vi "Save File RLT Panel File Name Setup.vi"(0 "File Locations In (Station A)":T4, 1 "Main Washer Control (Station A)":T6={"Appliance Details"={"FileVersionInfo"={"FileVersion"="", "ProductName"="", "InternalName"="", "CompanyName"="", "LegalCopyright"="", "FileDescription"=""}, "Dishwasher Info"={"Open Cup Weight (gm):"=0.0, "Auto Cup Weight (gm):"=0.0, "Detergent-Dish:"="", "Inlet Temperature-Dish:"="", "Cycle Mode-Dish:"="", "Unit Control-Dish:"="", "Manufacturer-Dish:"=""}, "Washer Info"={"Hot Water Temperature (Fahrenheit):"="", "Cold Water Temperature (Fahrenheit):"="", "Capacity (cu.ft):"=0.0, "Initial Cloth Weight:"=0.0, "Cloth Lot:"=0, "Model Family:"="", "Program Name:"="", "Cycle Selection:"="", "Wash Temperature:"="", "Rinse Temperature:"="", "Load Size:"=""}, "File Name Output Array"=[], "Calibration Output Array"=[], "Appliance Common"={"Engineer:"="", "Model Number:"="", "Serial Number:"="", "Comments:"="", "Station ID:"="", "Technician:"="", "TR Number:"="", "Lab ID:"="", "Voltage:"="", "Water Pressure (PSI):"="", "Test Date:"="", "Computer Name:"="", "IP Address:"="", "Ambient RH:"="", "Frequency:"="", "Build:"="", "Filename:"="", "Test Type:"="", "Load Run #:"=0, "Ambient Temperature (F):"="", "File Path:"=path "", "Cycles Per Year"=60}, "Water Heater"={"Heating Mode:"=""}, "Dryer"={"Heat Setting:"="", "Washer Water Temperature (60 ± 5°F):"=60, "Water Hardness (PPM):"=17, "Dryness Setting:"="", "Dryer Type:"="", "Exhaust:"="", "Drying Cycle:"="", "Load Type:"="", "Nominal Load Weight"="", "Dryer Initial IMC Data"={"Measured IMC (lbs)"=7.0, "Actual Initial RMC (%)"=7.0, "RMC (Desired %)"=100.0, "Bone Dry Wt(lbs)"=7.0, "Tolerance(%)"=5.0, "Actual Final RMC (%)"=7.0, "CEF (lbf/kWh)"=0.0, "Minimum Weight (lbf)"=0.0, "Average Weight (lbf)"=0.0, "Maximum Weight (lbf)"=0.0, "Measured IMC In Range?"=FALSE, "Moisture Reduction Factor"=55.5, "Field Use Factor"=1.04, "Empty Dryer Cold Weigth"=0.0, "Energy Standard"=enum."D2-Automatic Dryer", "Weight Cloth (lbs)"=0.0, "Relative Moisture Content (%)"=0.0, "Relative Moisture Content - Avg (%)"=0.0}}}, "Display Data (RLT)"={"Status Color"=0, "Serial Number Display"="", "Cycle Count Display"=0, "Station Label Display"="", "Current Run Start Time Display"=0.0, "Board ID Display"="", "RPM Display"=0, "Current Display"=0.0, "Current Path Display"=path "", "Saving Display"=FALSE, "Unit Type Display"=enum."", "Total Time On Display"=0.0, "UI Button"=FALSE}} {"Display Data (RLT)"."Current Display" format="%.2f"; "Display Data (RLT)"."Cycle Count Display" format="%04d"; "Appliance Details"."Dryer"."Dryer Initial IMC Data"."Maximum Weight (lbf)" format="%03_6g"; "Appliance Details"."Dryer"."Dryer Initial IMC Data"."Average Weight (lbf)" format="%03_6g"; "Appliance Details"."Dryer"."Dryer Initial IMC Data"."Minimum Weight (lbf)" format="%03_6g"; "Appliance Details"."Dryer"."Dryer Initial IMC Data"."CEF (lbf/kWh)" format="%03_6g"; "Appliance Details"."Dryer"."Dryer Initial IMC Data"."Actual Final RMC (%)" format="%03_6g"; "Appliance Details"."Dryer"."Dryer Initial IMC Data"."Tolerance(%)" format="%0#_6g"; "Appliance Details"."Dryer"."Dryer Initial IMC Data"."Bone Dry Wt(lbs)" format="%03_6g"; "Appliance Details"."Dryer"."Dryer Initial IMC Data"."RMC (Desired %)" format="%0#_6g"; "Appliance Details"."Dryer"."Dryer Initial IMC Data"."Actual Initial RMC (%)" format="%03_6g"; "Appliance Details"."Dryer"."Dryer Initial IMC Data"."Measured IMC (lbs)" format="%0#_6g"}, 5 "error in":errorcluster, 6 "RLT Station Type":T13, 11 "Front Panel (Station A)":T2={"Serial Number"="", "Lab ID"="", "TR Number"="", "Unit Type"=enum."", "Source"=228, "Address"=35} {"Address" format="%x"; "Source" format="%x"}) -> (12 "Active Stations":bool[](array[boolean]), 14 "File Locations Out":T4[](array[typedef]), 15 "Main Washer Controls Out":T6[](array[typedef]) {"Display Data (RLT)"."Current Display" format="%.2f"; "Display Data (RLT)"."Cycle Count Display" format="%04d"; "Appliance Details"."Dryer"."Dryer Initial IMC Data"."Maximum Weight (lbf)" format="%03_6g"; "Appliance Details"."Dryer"."Dryer Initial IMC Data"."Average Weight (lbf)" format="%03_6g"; "Appliance Details"."Dryer"."Dryer Initial IMC Data"."Minimum Weight (lbf)" format="%03_6g"; "Appliance Details"."Dryer"."Dryer Initial IMC Data"."CEF (lbf/kWh)" format="%03_6g"; "Appliance Details"."Dryer"."Dryer Initial IMC Data"."Actual Final RMC (%)" format="%03_6g"; "Appliance Details"."Dryer"."Dryer Initial IMC Data"."Tolerance(%)" format="%0#_6g"; "Appliance Details"."Dryer"."Dryer Initial IMC Data"."Bone Dry Wt(lbs)" format="%03_6g"; "Appliance Details"."Dryer"."Dryer Initial IMC Data"."RMC (Desired %)" format="%0#_6g"; "Appliance Details"."Dryer"."Dryer Initial IMC Data"."Actual Initial RMC (%)" format="%03_6g"; "Appliance Details"."Dryer"."Dryer Initial IMC Data"."Measured IMC (lbs)" format="%0#_6g"}, 19 "error out":errorcluster)   [LabVIEW 2016]
uses:
  Public/Type Definitions/Save File Unit Type.ctl
  Save File.lvlib
  Washer HCC/Washer HCC NEWFI/Type Definitions/HCC Filename Setup.ctl
  Type Definition/Save File DOE Data Save Filepaths.ctl
  File Setup.lvlib
  Type Definition/Save File DOE File Path Control.ctl
  <vilib>/Platform/fileVersionInfo.llb/FileVersionInformation.ctl
  Custom Pallet Controls/Custom Pallet String.ctl
  Type Definition/Save File DISH Dishwasher Details.ctl
  Public/Type Definitions/Save File Washer.ctl
  Type Definition/Save File RLT Station Type.ctl
  Public/Type Definitions/Save File Appliance Display.ctl
  Type Definition/DPT IMC Data.ctl
  Washer DOE/Type Definitions/DOE Appliance Common.ctl
  Washer DOE/Type Definitions/DOE Dryer Standard.ctl
panel:
  in  "Station D":T1="StationD"
  in  "Station C":T1="StationC"
  in  "Station B":T1="StationB"
  in  "Station A":T1="StationA"
  in  "Station D Check":bool
  in  "Station C Check":bool
  in  "Station B Check":bool
  in  "Station A Check":bool
  in  "Read Previous (Station D)":bool
  in  "Front Panel (Station D)":T2={"Serial Number"="", "Lab ID"="", "TR Number"="", "Unit Type"=enum."", "Source"=228, "Address"=35} {"Address" format="%x"; "Source" format="%x"}
  in  "Read Previous (Station C)":bool
  in  "Front Panel (Station C)":T2={"Serial Number"="", "Lab ID"="", "TR Number"="", "Unit Type"=enum."", "Source"=228, "Address"=35} {"Address" format="%x"; "Source" format="%x"}
  in  "Read Previous (Station B)":bool
  in  "Front Panel (Station B)":T2={"Serial Number"="", "Lab ID"="", "TR Number"="", "Unit Type"=enum."", "Source"=228, "Address"=35} {"Address" format="%x"; "Source" format="%x"}
  in  "Tab Control":enum32{"Page 1", "Page 2"}(tab)
  in  "File Locations In (Station D)":T4
  in  "File Locations In (Station C)":T4
  in  "File Locations In (Station B)":T4
  in  "Main Washer Control (Station D)":T6={"Appliance Details"={"FileVersionInfo"={"FileVersion"="", "ProductName"="", "InternalName"="", "CompanyName"="", "LegalCopyright"="", "FileDescription"=""}, "Dishwasher Info"={"Open Cup Weight (gm):"=0.0, "Auto Cup Weight (gm):"=0.0, "Detergent-Dish:"="", "Inlet Temperature-Dish:"="", "Cycle Mode-Dish:"="", "Unit Control-Dish:"="", "Manufacturer-Dish:"=""}, "Washer Info"={"Hot Water Temperature (Fahrenheit):"="", "Cold Water Temperature (Fahrenheit):"="", "Capacity (cu.ft):"=0.0, "Initial Cloth Weight:"=0.0, "Cloth Lot:"=0, "Model Family:"="", "Program Name:"="", "Cycle Selection:"="", "Wash Temperature:"="", "Rinse Temperature:"="", "Load Size:"=""}, "File Name Output Array"=[], "Calibration Output Array"=[], "Appliance Common"={"Engineer:"="", "Model Number:"="", "Serial Number:"="", "Comments:"="", "Station ID:"="", "Technician:"="", "TR Number:"="", "Lab ID:"="", "Voltage:"="", "Water Pressure (PSI):"="", "Test Date:"="", "Computer Name:"="", "IP Address:"="", "Ambient RH:"="", "Frequency:"="", "Build:"="", "Filename:"="", "Test Type:"="", "Load Run #:"=0, "Ambient Temperature (F):"="", "File Path:"=path "", "Cycles Per Year"=60}, "Water Heater"={"Heating Mode:"=""}, "Dryer"={"Heat Setting:"="", "Washer Water Temperature (60 ± 5°F):"=60, "Water Hardness (PPM):"=17, "Dryness Setting:"="", "Dryer Type:"="", "Exhaust:"="", "Drying Cycle:"="", "Load Type:"="", "Nominal Load Weight"="", "Dryer Initial IMC Data"={"Measured IMC (lbs)"=7.0, "Actual Initial RMC (%)"=7.0, "RMC (Desired %)"=100.0, "Bone Dry Wt(lbs)"=7.0, "Tolerance(%)"=5.0, "Actual Final RMC (%)"=7.0, "CEF (lbf/kWh)"=0.0, "Minimum Weight (lbf)"=0.0, "Average Weight (lbf)"=0.0, "Maximum Weight (lbf)"=0.0, "Measured IMC In Range?"=FALSE, "Moisture Reduction Factor"=55.5, "Field Use Factor"=1.04, "Empty Dryer Cold Weigth"=0.0, "Energy Standard"=enum."D2-Automatic Dryer", "Weight Cloth (lbs)"=0.0, "Relative Moisture Content (%)"=0.0, "Relative Moisture Content - Avg (%)"=0.0}}}, "Display Data (RLT)"={"Status Color"=0, "Serial Number Display"="", "Cycle Count Display"=0, "Station Label Display"="", "Current Run Start Time Display"=0.0, "Board ID Display"="", "RPM Display"=0, "Current Display"=0.0, "Current Path Display"=path "", "Saving Display"=FALSE, "Unit Type Display"=enum."", "Total Time On Display"=0.0, "UI Button"=FALSE}} {"Display Data (RLT)"."Current Display" format="%.2f"; "Display Data (RLT)"."Cycle Count Display" format="%04d"; "Appliance Details"."Dryer"."Dryer Initial IMC Data"."Maximum Weight (lbf)" format="%03_6g"; "Appliance Details"."Dryer"."Dryer Initial IMC Data"."Average Weight (lbf)" format="%03_6g"; "Appliance Details"."Dryer"."Dryer Initial IMC Data"."Minimum Weight (lbf)" format="%03_6g"; "Appliance Details"."Dryer"."Dryer Initial IMC Data"."CEF (lbf/kWh)" format="%03_6g"; "Appliance Details"."Dryer"."Dryer Initial IMC Data"."Actual Final RMC (%)" format="%03_6g"; "Appliance Details"."Dryer"."Dryer Initial IMC Data"."Tolerance(%)" format="%0#_6g"; "Appliance Details"."Dryer"."Dryer Initial IMC Data"."Bone Dry Wt(lbs)" format="%03_6g"; "Appliance Details"."Dryer"."Dryer Initial IMC Data"."RMC (Desired %)" format="%0#_6g"; "Appliance Details"."Dryer"."Dryer Initial IMC Data"."Actual Initial RMC (%)" format="%03_6g"; "Appliance Details"."Dryer"."Dryer Initial IMC Data"."Measured IMC (lbs)" format="%0#_6g"}
  in  "Main Washer Control (Station C)":T6={"Appliance Details"={"FileVersionInfo"={"FileVersion"="", "ProductName"="", "InternalName"="", "CompanyName"="", "LegalCopyright"="", "FileDescription"=""}, "Dishwasher Info"={"Open Cup Weight (gm):"=0.0, "Auto Cup Weight (gm):"=0.0, "Detergent-Dish:"="", "Inlet Temperature-Dish:"="", "Cycle Mode-Dish:"="", "Unit Control-Dish:"="", "Manufacturer-Dish:"=""}, "Washer Info"={"Hot Water Temperature (Fahrenheit):"="", "Cold Water Temperature (Fahrenheit):"="", "Capacity (cu.ft):"=0.0, "Initial Cloth Weight:"=0.0, "Cloth Lot:"=0, "Model Family:"="", "Program Name:"="", "Cycle Selection:"="", "Wash Temperature:"="", "Rinse Temperature:"="", "Load Size:"=""}, "File Name Output Array"=[], "Calibration Output Array"=[], "Appliance Common"={"Engineer:"="", "Model Number:"="", "Serial Number:"="", "Comments:"="", "Station ID:"="", "Technician:"="", "TR Number:"="", "Lab ID:"="", "Voltage:"="", "Water Pressure (PSI):"="", "Test Date:"="", "Computer Name:"="", "IP Address:"="", "Ambient RH:"="", "Frequency:"="", "Build:"="", "Filename:"="", "Test Type:"="", "Load Run #:"=0, "Ambient Temperature (F):"="", "File Path:"=path "", "Cycles Per Year"=60}, "Water Heater"={"Heating Mode:"=""}, "Dryer"={"Heat Setting:"="", "Washer Water Temperature (60 ± 5°F):"=60, "Water Hardness (PPM):"=17, "Dryness Setting:"="", "Dryer Type:"="", "Exhaust:"="", "Drying Cycle:"="", "Load Type:"="", "Nominal Load Weight"="", "Dryer Initial IMC Data"={"Measured IMC (lbs)"=7.0, "Actual Initial RMC (%)"=7.0, "RMC (Desired %)"=100.0, "Bone Dry Wt(lbs)"=7.0, "Tolerance(%)"=5.0, "Actual Final RMC (%)"=7.0, "CEF (lbf/kWh)"=0.0, "Minimum Weight (lbf)"=0.0, "Average Weight (lbf)"=0.0, "Maximum Weight (lbf)"=0.0, "Measured IMC In Range?"=FALSE, "Moisture Reduction Factor"=55.5, "Field Use Factor"=1.04, "Empty Dryer Cold Weigth"=0.0, "Energy Standard"=enum."D2-Automatic Dryer", "Weight Cloth (lbs)"=0.0, "Relative Moisture Content (%)"=0.0, "Relative Moisture Content - Avg (%)"=0.0}}}, "Display Data (RLT)"={"Status Color"=0, "Serial Number Display"="", "Cycle Count Display"=0, "Station Label Display"="", "Current Run Start Time Display"=0.0, "Board ID Display"="", "RPM Display"=0, "Current Display"=0.0, "Current Path Display"=path "", "Saving Display"=FALSE, "Unit Type Display"=enum."", "Total Time On Display"=0.0, "UI Button"=FALSE}} {"Display Data (RLT)"."Current Display" format="%.2f"; "Display Data (RLT)"."Cycle Count Display" format="%04d"; "Appliance Details"."Dryer"."Dryer Initial IMC Data"."Maximum Weight (lbf)" format="%03_6g"; "Appliance Details"."Dryer"."Dryer Initial IMC Data"."Average Weight (lbf)" format="%03_6g"; "Appliance Details"."Dryer"."Dryer Initial IMC Data"."Minimum Weight (lbf)" format="%03_6g"; "Appliance Details"."Dryer"."Dryer Initial IMC Data"."CEF (lbf/kWh)" format="%03_6g"; "Appliance Details"."Dryer"."Dryer Initial IMC Data"."Actual Final RMC (%)" format="%03_6g"; "Appliance Details"."Dryer"."Dryer Initial IMC Data"."Tolerance(%)" format="%0#_6g"; "Appliance Details"."Dryer"."Dryer Initial IMC Data"."Bone Dry Wt(lbs)" format="%03_6g"; "Appliance Details"."Dryer"."Dryer Initial IMC Data"."RMC (Desired %)" format="%0#_6g"; "Appliance Details"."Dryer"."Dryer Initial IMC Data"."Actual Initial RMC (%)" format="%03_6g"; "Appliance Details"."Dryer"."Dryer Initial IMC Data"."Measured IMC (lbs)" format="%0#_6g"}
  in  "Main Washer Control (Station B)":T6={"Appliance Details"={"FileVersionInfo"={"FileVersion"="", "ProductName"="", "InternalName"="", "CompanyName"="", "LegalCopyright"="", "FileDescription"=""}, "Dishwasher Info"={"Open Cup Weight (gm):"=0.0, "Auto Cup Weight (gm):"=0.0, "Detergent-Dish:"="", "Inlet Temperature-Dish:"="", "Cycle Mode-Dish:"="", "Unit Control-Dish:"="", "Manufacturer-Dish:"=""}, "Washer Info"={"Hot Water Temperature (Fahrenheit):"="", "Cold Water Temperature (Fahrenheit):"="", "Capacity (cu.ft):"=0.0, "Initial Cloth Weight:"=0.0, "Cloth Lot:"=0, "Model Family:"="", "Program Name:"="", "Cycle Selection:"="", "Wash Temperature:"="", "Rinse Temperature:"="", "Load Size:"=""}, "File Name Output Array"=[], "Calibration Output Array"=[], "Appliance Common"={"Engineer:"="", "Model Number:"="", "Serial Number:"="", "Comments:"="", "Station ID:"="", "Technician:"="", "TR Number:"="", "Lab ID:"="", "Voltage:"="", "Water Pressure (PSI):"="", "Test Date:"="", "Computer Name:"="", "IP Address:"="", "Ambient RH:"="", "Frequency:"="", "Build:"="", "Filename:"="", "Test Type:"="", "Load Run #:"=0, "Ambient Temperature (F):"="", "File Path:"=path "", "Cycles Per Year"=60}, "Water Heater"={"Heating Mode:"=""}, "Dryer"={"Heat Setting:"="", "Washer Water Temperature (60 ± 5°F):"=60, "Water Hardness (PPM):"=17, "Dryness Setting:"="", "Dryer Type:"="", "Exhaust:"="", "Drying Cycle:"="", "Load Type:"="", "Nominal Load Weight"="", "Dryer Initial IMC Data"={"Measured IMC (lbs)"=7.0, "Actual Initial RMC (%)"=7.0, "RMC (Desired %)"=100.0, "Bone Dry Wt(lbs)"=7.0, "Tolerance(%)"=5.0, "Actual Final RMC (%)"=7.0, "CEF (lbf/kWh)"=0.0, "Minimum Weight (lbf)"=0.0, "Average Weight (lbf)"=0.0, "Maximum Weight (lbf)"=0.0, "Measured IMC In Range?"=FALSE, "Moisture Reduction Factor"=55.5, "Field Use Factor"=1.04, "Empty Dryer Cold Weigth"=0.0, "Energy Standard"=enum."D2-Automatic Dryer", "Weight Cloth (lbs)"=0.0, "Relative Moisture Content (%)"=0.0, "Relative Moisture Content - Avg (%)"=0.0}}}, "Display Data (RLT)"={"Status Color"=0, "Serial Number Display"="", "Cycle Count Display"=0, "Station Label Display"="", "Current Run Start Time Display"=0.0, "Board ID Display"="", "RPM Display"=0, "Current Display"=0.0, "Current Path Display"=path "", "Saving Display"=FALSE, "Unit Type Display"=enum."", "Total Time On Display"=0.0, "UI Button"=FALSE}} {"Display Data (RLT)"."Current Display" format="%.2f"; "Display Data (RLT)"."Cycle Count Display" format="%04d"; "Appliance Details"."Dryer"."Dryer Initial IMC Data"."Maximum Weight (lbf)" format="%03_6g"; "Appliance Details"."Dryer"."Dryer Initial IMC Data"."Average Weight (lbf)" format="%03_6g"; "Appliance Details"."Dryer"."Dryer Initial IMC Data"."Minimum Weight (lbf)" format="%03_6g"; "Appliance Details"."Dryer"."Dryer Initial IMC Data"."CEF (lbf/kWh)" format="%03_6g"; "Appliance Details"."Dryer"."Dryer Initial IMC Data"."Actual Final RMC (%)" format="%03_6g"; "Appliance Details"."Dryer"."Dryer Initial IMC Data"."Tolerance(%)" format="%0#_6g"; "Appliance Details"."Dryer"."Dryer Initial IMC Data"."Bone Dry Wt(lbs)" format="%03_6g"; "Appliance Details"."Dryer"."Dryer Initial IMC Data"."RMC (Desired %)" format="%0#_6g"; "Appliance Details"."Dryer"."Dryer Initial IMC Data"."Actual Initial RMC (%)" format="%03_6g"; "Appliance Details"."Dryer"."Dryer Initial IMC Data"."Measured IMC (lbs)" format="%0#_6g"}
  in  "Read Previous (Station A)":bool
  in  "Tab Control 2":enum32{"Input Data", "Error Data"}(tab)
  in  "Complete":bool
  # "OR"
  # "OR"
  # "OR"
  # "OR"
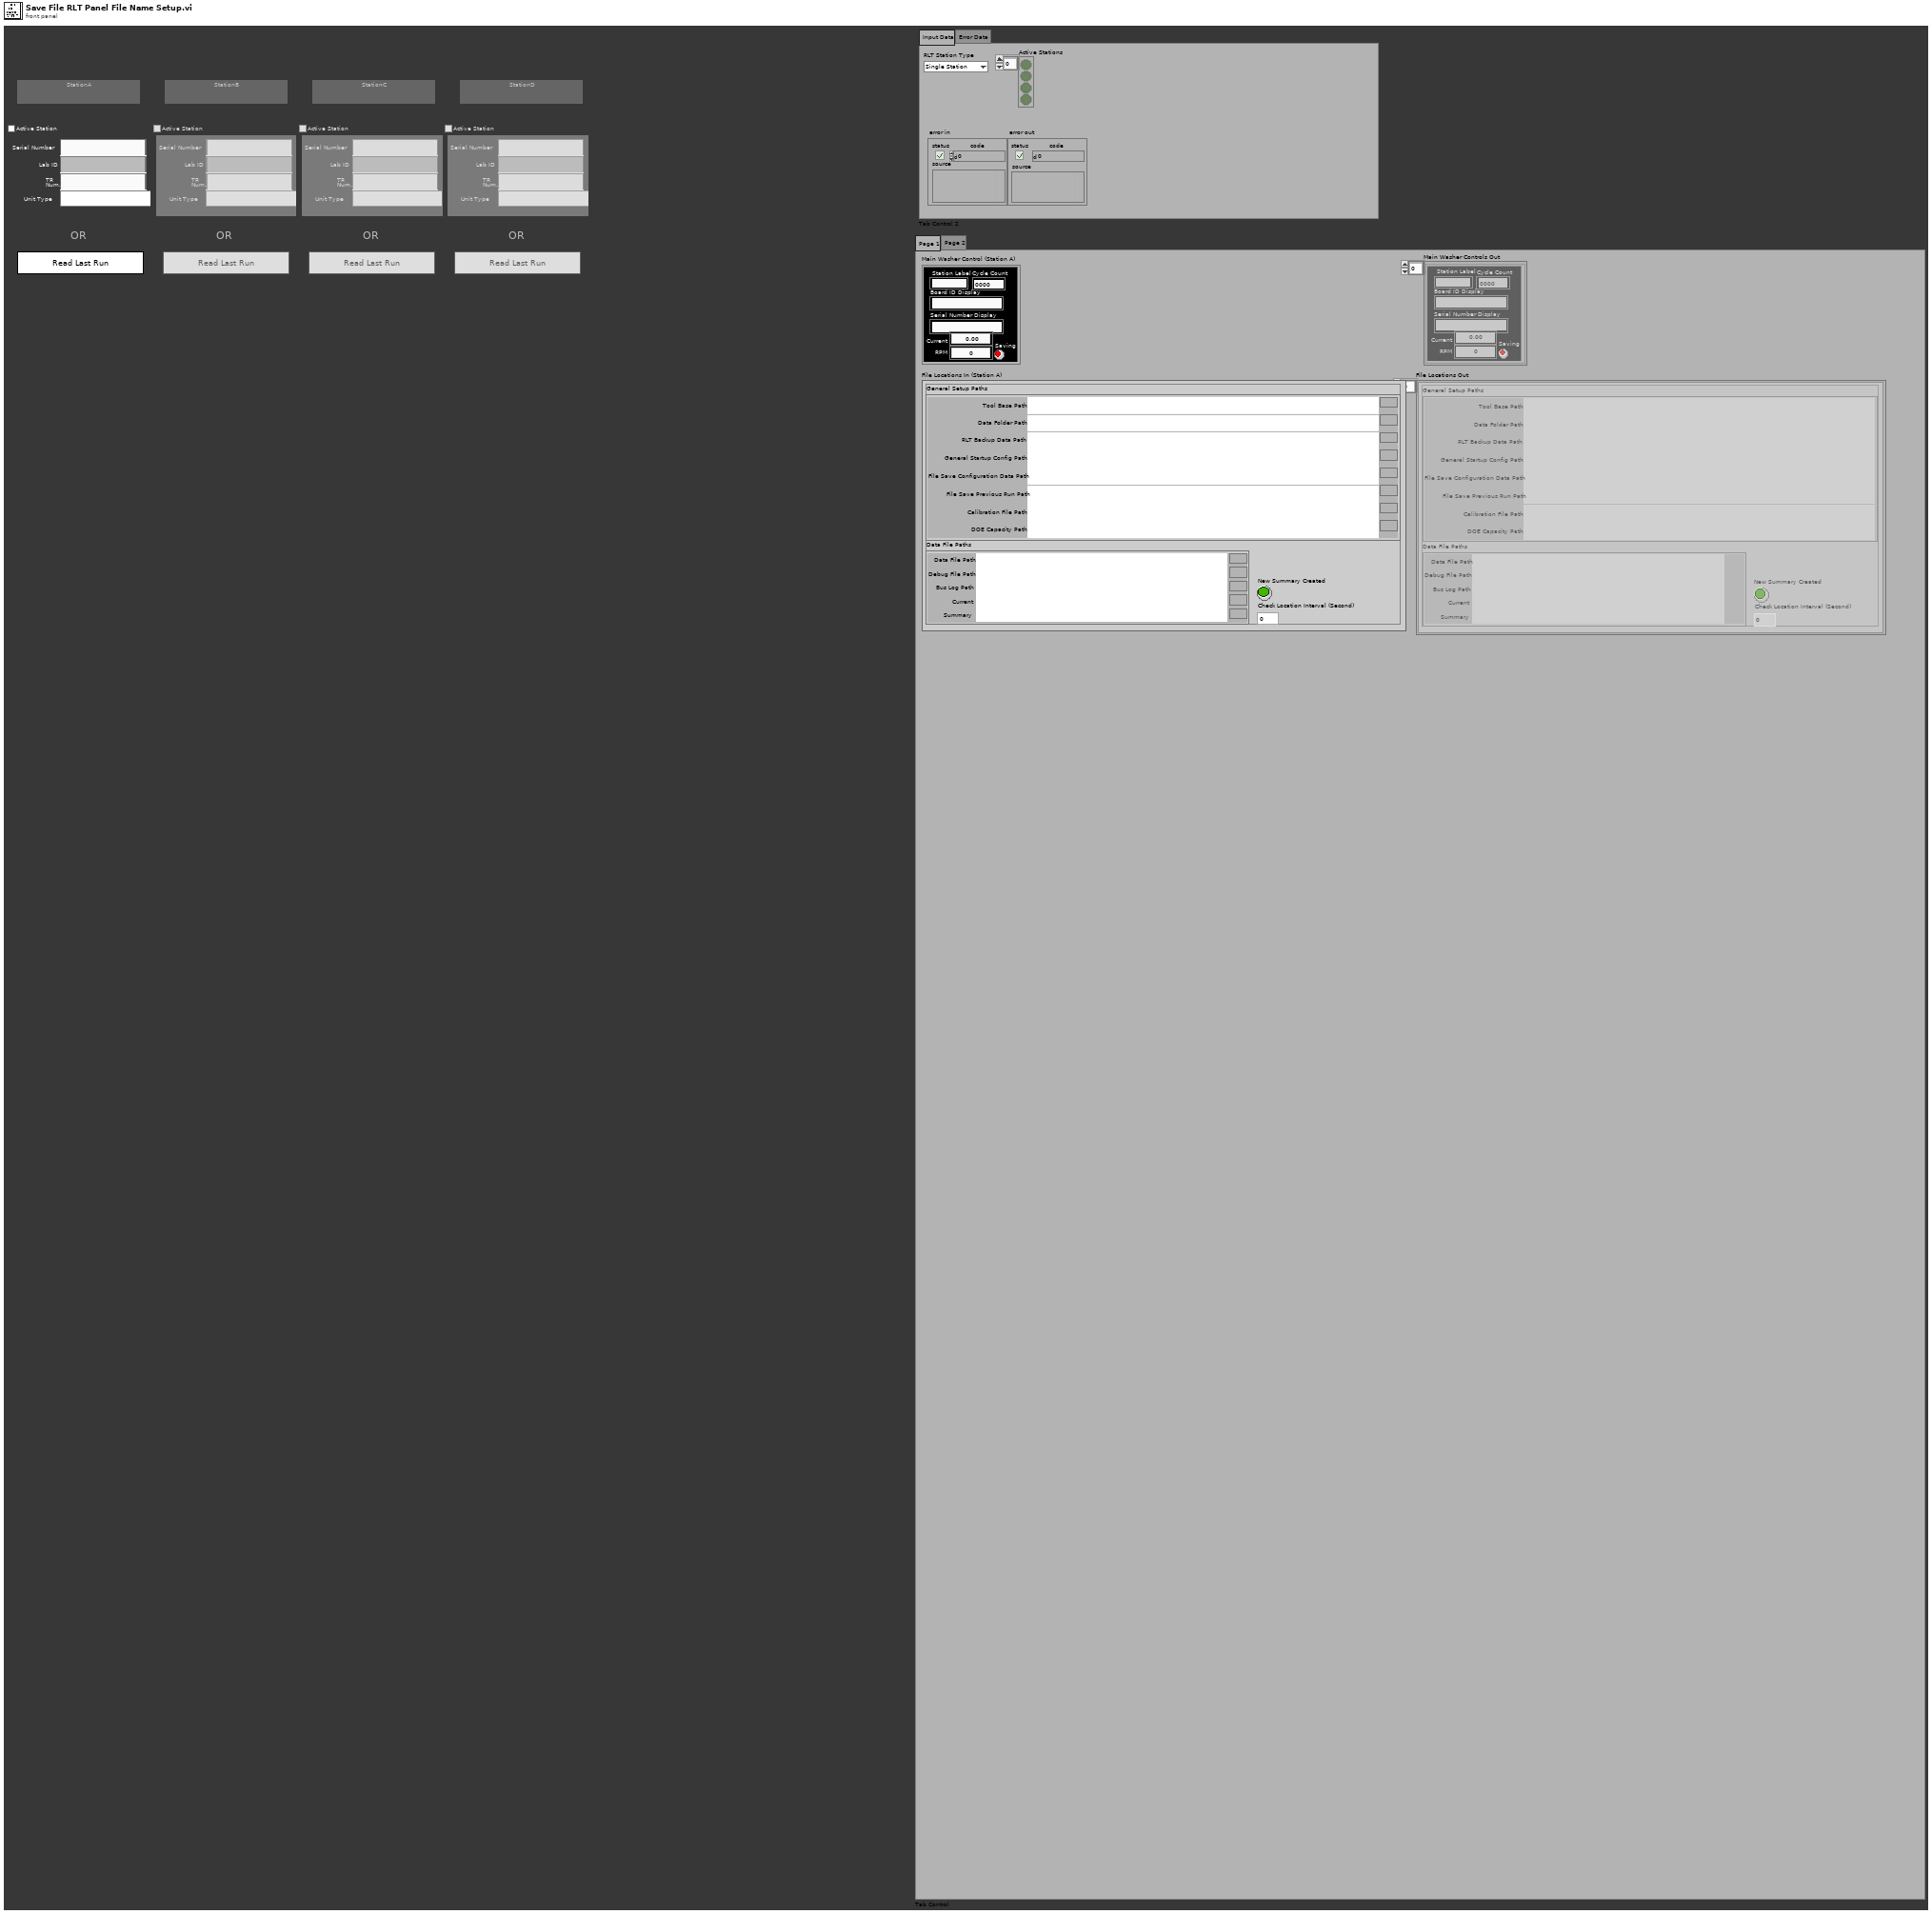
[diagram p1: front panel]
types:
  T1 = typedef "Custom Pallet String.ctl" = string
  T2 = typedef "HCC Filename Setup.ctl" = cluster{"Serial Number":string, "Lab ID":string, "TR Number":string, "Unit Type":T3, "Source":u8, "Address":u8}
  T3 = typedef "Save File.lvlib/Save File Unit Type.ctl" = enum32{"", "Viper", "Hawk", "2015"}
  T4 = typedef "File Setup.lvlib/Save File DOE File Path Control.ctl" = cluster{"General Setup Paths":cluster{"Calibration File Path":path, "DOE Capacity Path":path, "Data Folder Path":path, "RLT Backup Data Path":path, "Tool Base Path":path, "General Startup Config Path":path, "File Save Previous Run Path":path, "File Save Configuration Data Path":path}, "Data File Paths":T5, "New Summary Created":bool, "Check Location Interval (Second)":i32}
  T5 = typedef "File Setup.lvlib/Save File DOE Data Save Filepaths.ctl" = cluster{"Data File Path":path, "Debug File Path":path, "Bus Log Path":path, "Current":path, "Summary":path}
  T6 = typedef "Save File.lvlib/Save File Washer.ctl" = cluster{"Appliance Details":T7, "Display Data (RLT)":T12}
  T7 = typedef "File Setup.lvlib/Save File DISH Dishwasher Details.ctl" = cluster{"FileVersionInfo":T8, "Dishwasher Info":cluster{"Open Cup Weight (gm):":dbl, "Auto Cup Weight (gm):":dbl, "Detergent-Dish:":string, "Inlet Temperature-Dish:":string, "Cycle Mode-Dish:":string, "Unit Control-Dish:":string, "Manufacturer-Dish:":string}, "Washer Info":cluster{"Hot Water Temperature (Fahrenheit):":string, "Cold Water Temperature (Fahrenheit):":string, "Capacity (cu.ft):":dbl, "Initial Cloth Weight:":dbl, "Cloth Lot:":i32, "Model Family:":string, "Program Name:":string, "Cycle Selection:":string, "Wash Temperature:":string, "Rinse Temperature:":string, "Load Size:":string}, "File Name Output Array":string[][], "Calibration Output Array":string[][], "Appliance Common":T9, "Water Heater":cluster{"Heating Mode:":string}, "Dryer":cluster{"Heat Setting:":T1, "Washer Water Temperature (60 ± 5°F):":u16, "Water Hardness (PPM):":u16, "Dryness Setting:":T1, "Dryer Type:":string, "Exhaust:":string, "Drying Cycle:":string, "Load Type:":string, "Nominal Load Weight":string, "Dryer Initial IMC Data":T10}}
  T8 = typedef "FileVersionInformation.ctl" = cluster{"FileVersion":string, "ProductName":string, "InternalName":string, "CompanyName":string, "LegalCopyright":string, "FileDescription":string}
  T9 = typedef "DOE Appliance Common.ctl" = cluster{"Engineer:":string, "Model Number:":string, "Serial Number:":string, "Comments:":string, "Station ID:":string, "Technician:":string, "TR Number:":string, "Lab ID:":string, "Voltage:":string, "Water Pressure (PSI):":string, "Test Date:":string, "Computer Name:":string, "IP Address:":string, "Ambient RH:":string, "Frequency:":string, "Build:":string, "Filename:":string, "Test Type:":string, "Load Run #:":i32, "Ambient Temperature (F):":string, "File Path:":path, "Cycles Per Year":u32}
  T10 = typedef "DPT IMC Data.ctl" = cluster{"Measured IMC (lbs)":dbl, "Actual Initial RMC (%)":dbl, "RMC (Desired %)":dbl, "Bone Dry Wt(lbs)":dbl, "Tolerance(%)":dbl, "Actual Final RMC (%)":dbl, "CEF (lbf/kWh)":dbl, "Minimum Weight (lbf)":dbl, "Average Weight (lbf)":dbl, "Maximum Weight (lbf)":dbl, "Measured IMC In Range?":bool, "Moisture Reduction Factor":dbl, "Field Use Factor":dbl, "Empty Dryer Cold Weigth":dbl, "Energy Standard":T11, "Weight Cloth (lbs)":dbl, "Relative Moisture Content (%)":dbl, "Relative Moisture Content - Avg (%)":dbl}
  T11 = typedef "DOE Dryer Standard.ctl" = enum16{"D2-Automatic Dryer", "D2-Timer Dryer", "D1-Automatic Dryer", "D1-Timer Dryer", "Other"}
  T12 = typedef "Save File Appliance Display.ctl" = cluster{"Status Color":u32, "Serial Number Display":string, "Cycle Count Display":i32, "Station Label Display":string, "Current Run Start Time Display":dbl, "Board ID Display":string, "RPM Display":u32, "Current Display":dbl, "Current Path Display":path, "Saving Display":bool, "Unit Type Display":T3, "Total Time On Display":dbl, "UI Button":bool}
  T13 = typedef "Save File RLT Station Type.ctl" = enum16{"Single Station", "Four Stations"}
  T14 = enum8{"Enabled", "Disabled", "Disabled and Grayed Out"}
  T15 = enum32{"invalid app kind", "Development System", "Run Time System", "Student Edition", "Embedded LabVIEW", "Evaluation", "Custom"}
  T16 = enum32{"Invalid", "Standard", "Closed", "Hidden", "Minimized", "Maximized"}
  T17 = cluster{"Core":cluster{"Current VI Reference":refnum<vi>, "Close Panel on Exit?":bool}, "Main Washer Control (Station A)":T6, "Main Washer Control (Station B)":T6, "Main Washer Control (Station C)":T6, "Main Washer Control (Station D)":T6, "Front Panel (Station A)":T2, "Front Panel (Station B)":T2, "Front Panel (Station C)":T2, "Front Panel (Station D)":T2, "File Locations In (Station A)":T4, "File Locations In (Station B)":T4, "File Locations In (Station C)":T4, "File Locations In (Station D)":T4, "Active Stations":bool[], "RLT Station Type":T13}
  T18 = cluster{"Current VI Reference":refnum<vi>, "Close Panel on Exit?":bool}
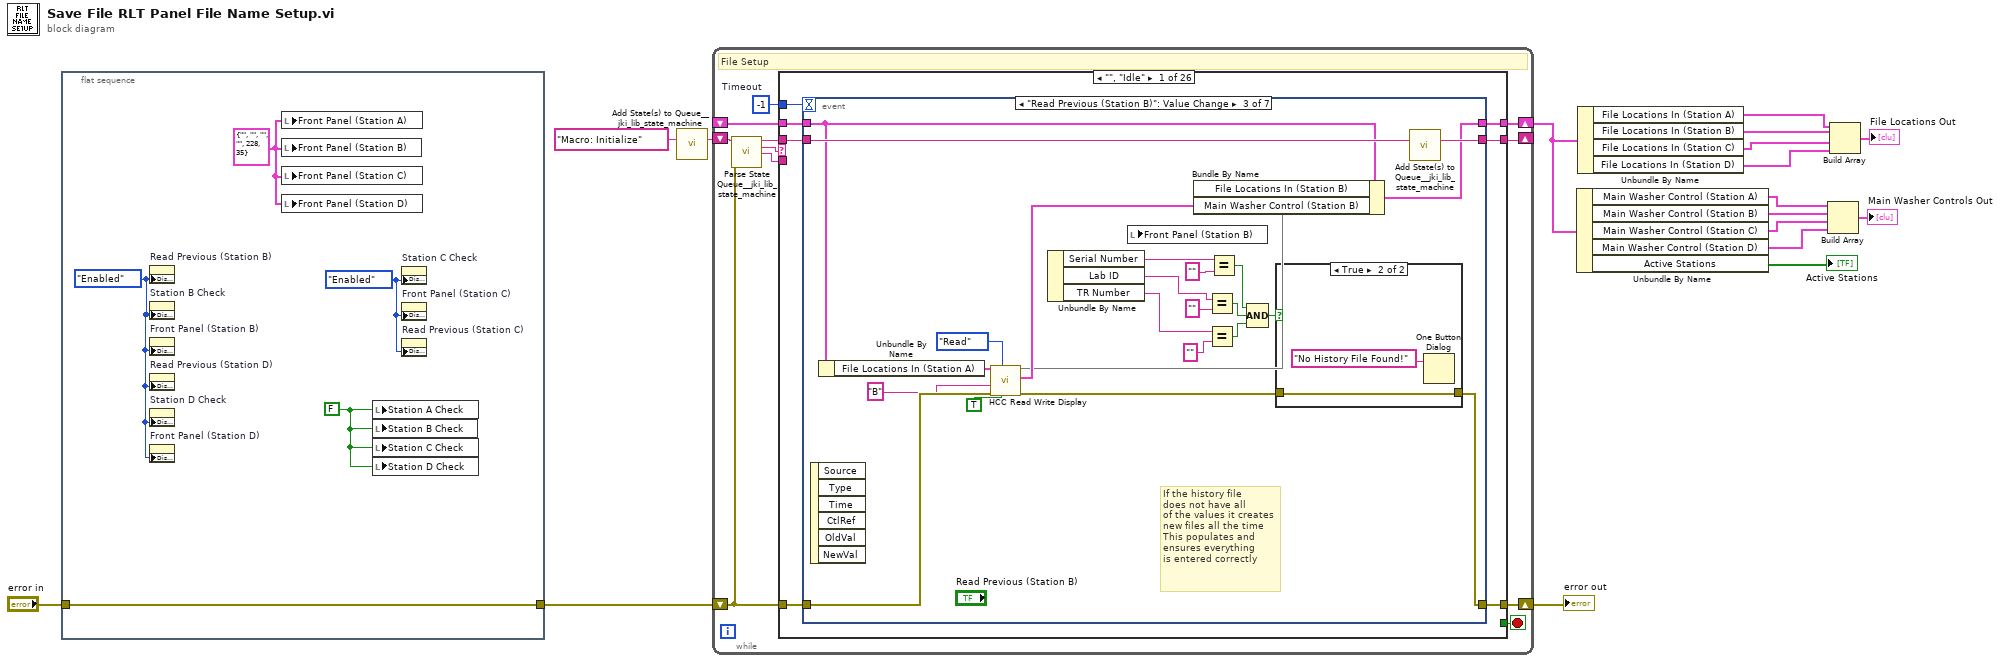
[diagram p0: block diagram]
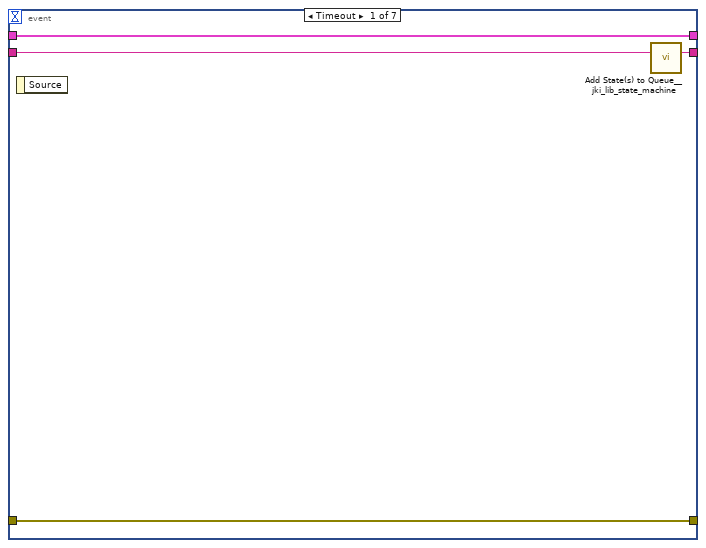
[diagram p2: hidden frame]
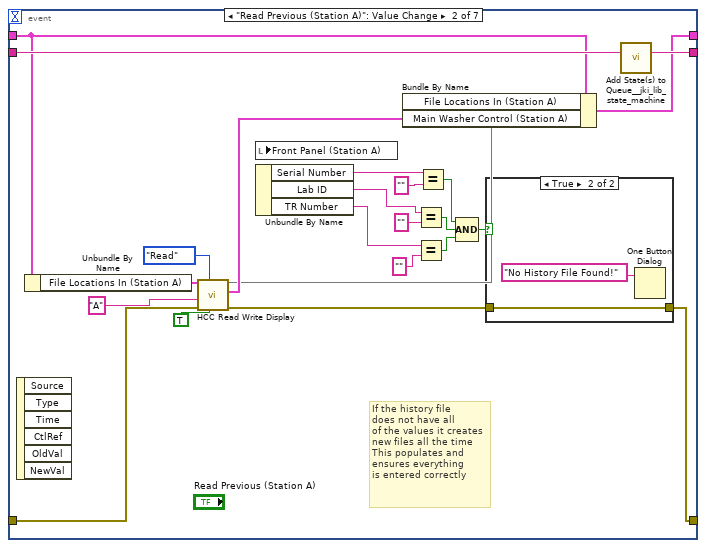
[diagram p3: hidden frame]
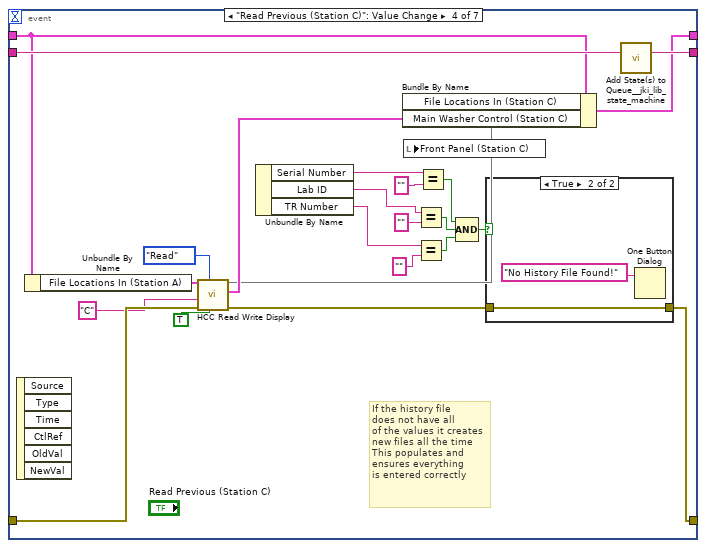
[diagram p6: hidden frame]
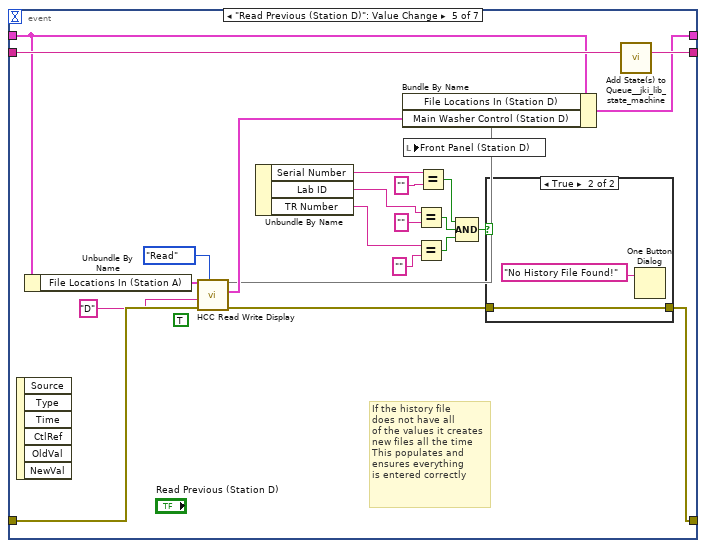
[diagram p8: hidden frame]
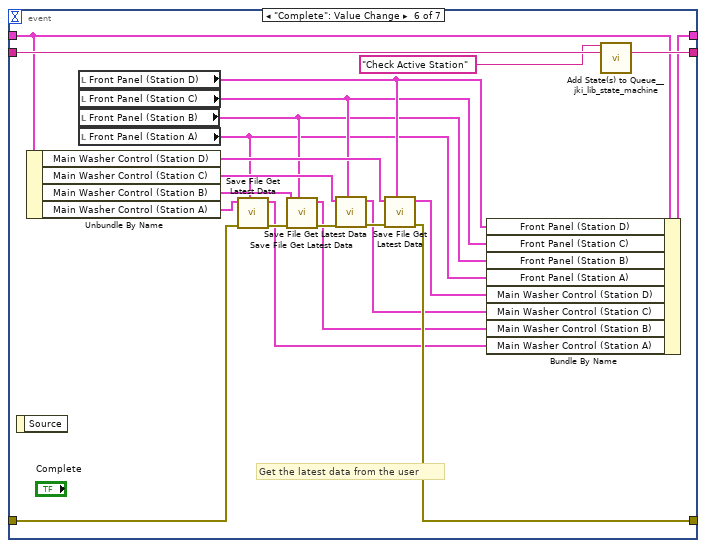
[diagram p10: hidden frame]
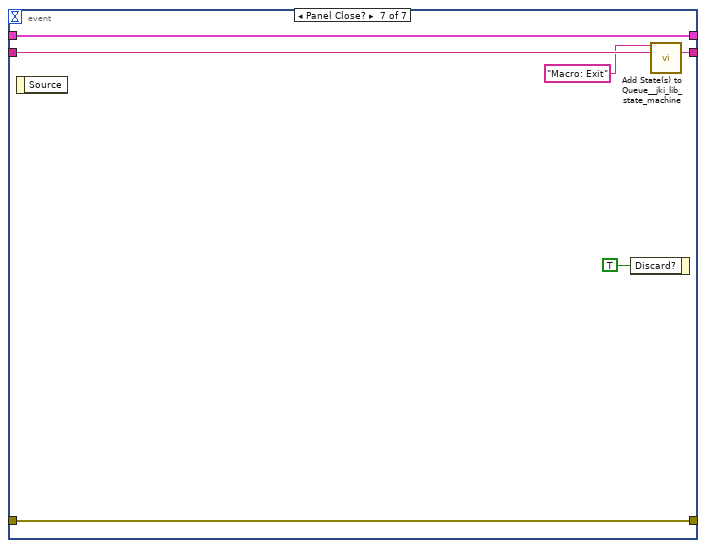
[diagram p11: hidden frame]
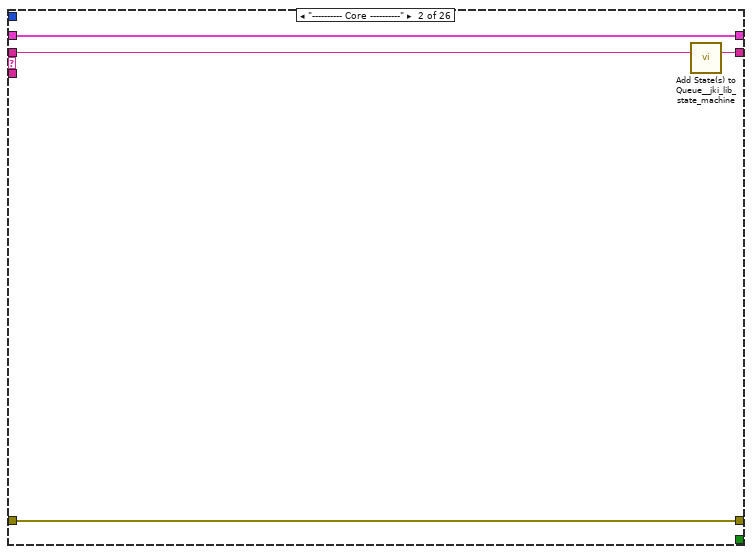
[diagram p12: hidden frame]
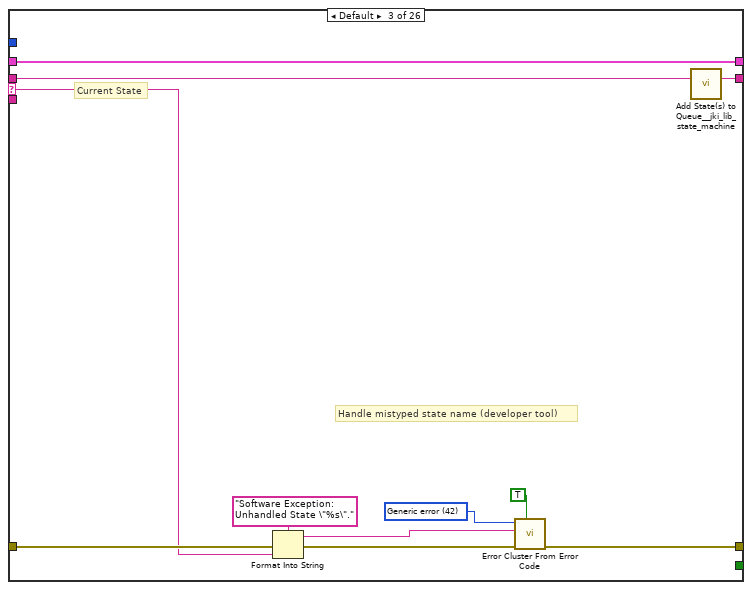
[diagram p13: hidden frame]
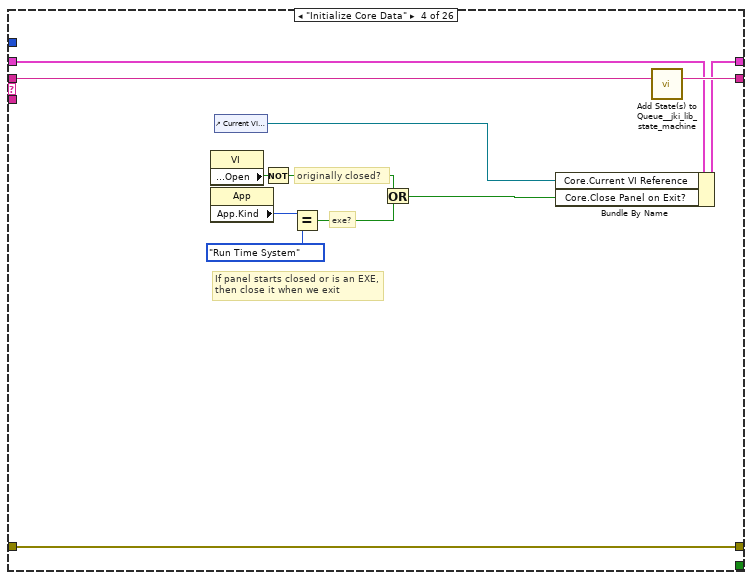
[diagram p14: hidden frame]
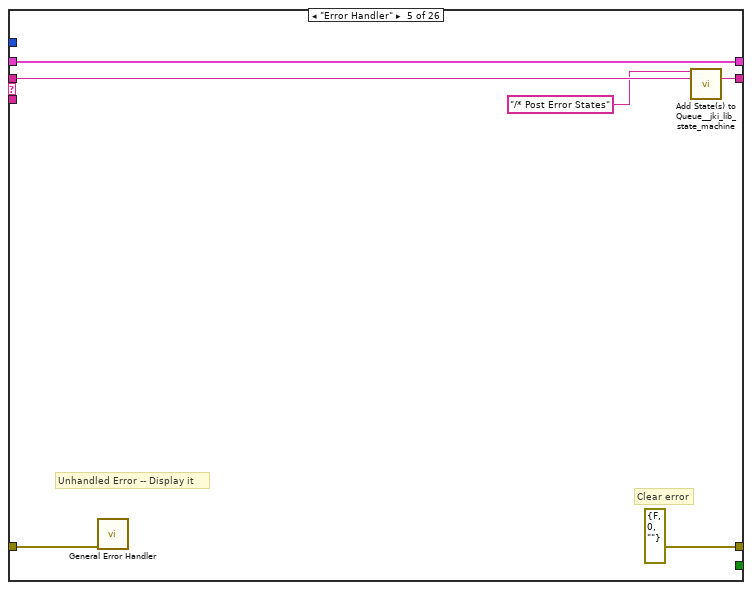
[diagram p15: hidden frame]
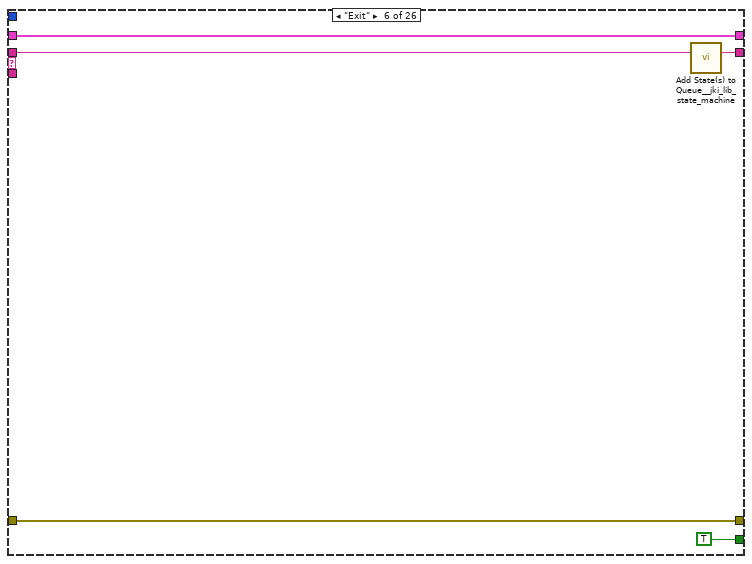
[diagram p16: hidden frame]
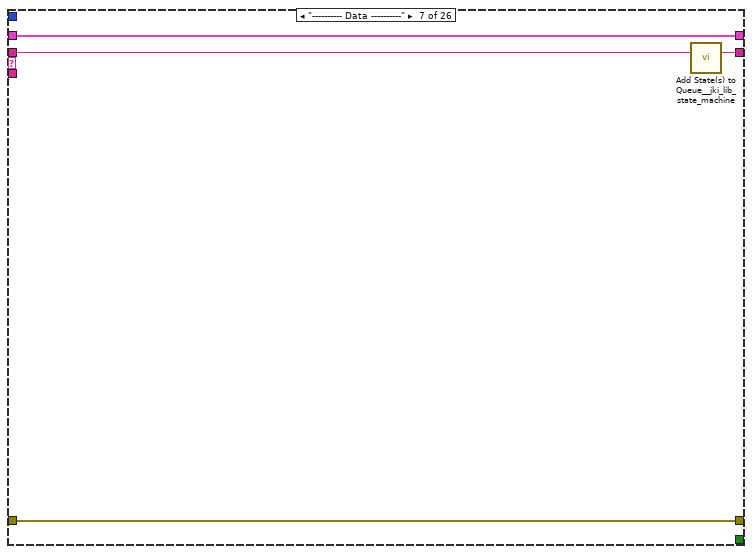
[diagram p17: hidden frame]
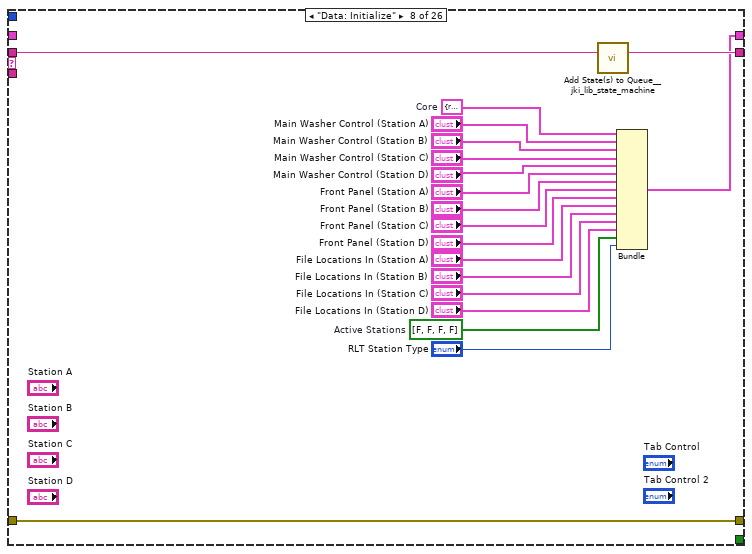
[diagram p18: hidden frame]
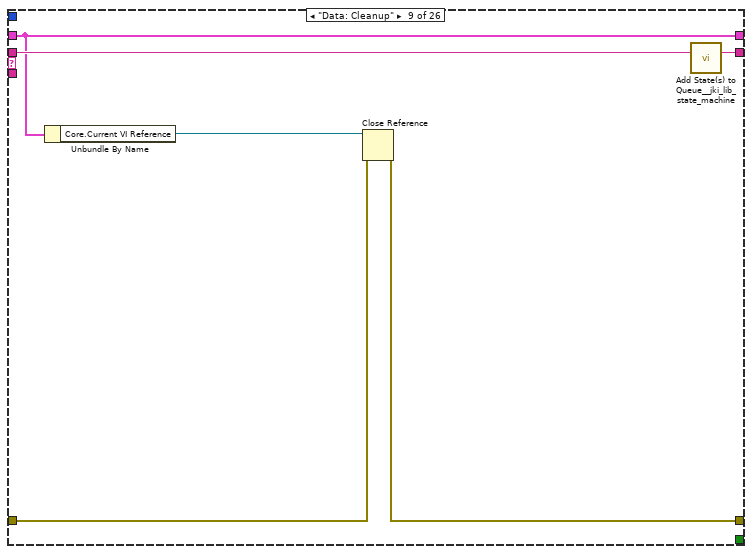
[diagram p19: hidden frame]
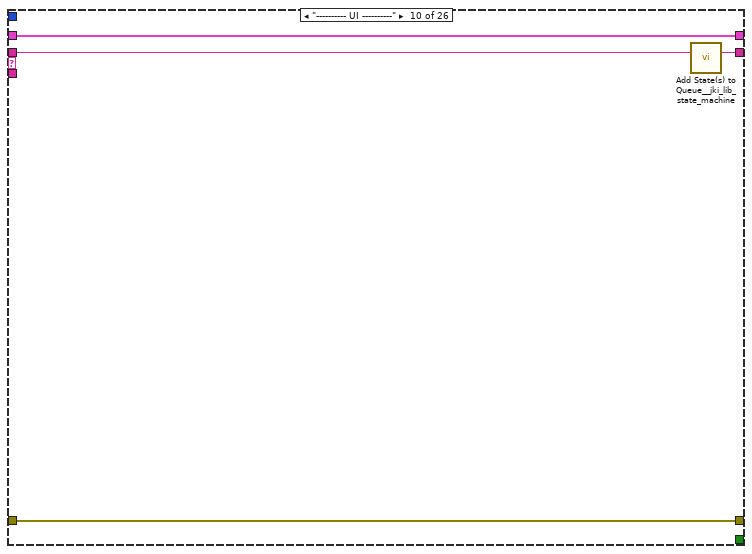
[diagram p20: hidden frame]
diagram:
  n1 = flat-sequence {
    tunnel: "error in" -> [w20]
    tunnel: [w20] -> w2
    frame #0 {
      w18 = T2 {"Serial Number"="", "Lab ID"="", "TR Number"="", "Unit Type"=enum."", "Source"=228, "Address"=35} ("Front Panel (Station A)")
      w19 = FALSE ("Station A Check")
      w22 = T14."Enabled" ("Disabled")
      w21 = T14."Enabled" ("Disabled")
      n2 = property on="Read Previous (Station B)" class="Bool"("DisabledEnum"=w21) -> ()  [unwired: 2 in, 2 out]
      n3 = property on="Station B Check" class="Bool (strict)"("DisabledEnum"=w21) -> ()  [unwired: 2 in, 2 out]
      n4 = property on="Front Panel (Station B)" class="Clust (strict)"("DisabledEnum"=w21) -> ()  [unwired: 2 in, 2 out]
      n5 = property on="Read Previous (Station D)" class="Bool"("DisabledEnum"=w21) -> ()  [unwired: 2 in, 2 out]
      n6 = property on="Station D Check" class="Bool (strict)"("DisabledEnum"=w21) -> ()  [unwired: 2 in, 2 out]
      n7 = property on="Front Panel (Station D)" class="Clust (strict)"("DisabledEnum"=w21) -> ()  [unwired: 2 in, 2 out]
      n8 = local write "Front Panel (Station A)"(w18) -> ()
      n9 = local write "Front Panel (Station B)"(w18) -> ()
      n10 = local write "Front Panel (Station C)"(w18) -> ()
      n11 = local write "Front Panel (Station D)"(w18) -> ()
      n12 = local write "Station A Check"(w19) -> ()
      n13 = local write "Station B Check"(w19) -> ()
      n14 = local write "Station C Check"(w19) -> ()
      n15 = local write "Station D Check"(w19) -> ()
      n16 = property on="Station C Check" class="Bool (strict)"("DisabledEnum"=w22) -> ()  [unwired: 2 in, 2 out]
      n17 = property on="Front Panel (Station C)" class="Clust (strict)"("DisabledEnum"=w22) -> ()  [unwired: 2 in, 2 out]
      n18 = property on="Read Previous (Station C)" class="Bool"("DisabledEnum"=w22) -> ()  [unwired: 2 in, 2 out]
    }
  }
  n19 = call <vilib>:"Add State(s) to Queue__jki_lib_state_machine.vi"("State(s) in (\"\")"="Macro: Initialize") -> ("States Out"=w17:string)  [unwired: 14 in]
  n20 = while "File Setup" {
    shift-right: [w26] -> w14
    shift-left: _ -> [w25]
    shift-right: [w29] -> w16
    shift-left: w2 -> [w23]
    shift-right: [w28] -> _
    shift-left: w17 -> [w30]
    stop <- w27 stop-if-true
    w24 = -1  # Timeout
    # "File Setup"
    n21 = call <vilib>:"Parse State Queue__jki_lib_state_machine.vi"("State Queue"=w30, "Error In (no error)"=w23) -> ("Remaining States"=w32:string, "Current State"=w33:string, "Arguments"=w31:string)  [unwired: 11 in]
    n22 = case shown="\"\", \"Idle\"" w33 {
      selector: w33 -> [_ _ w180 _ _ _ _ _ _ _ _ _ _ _ _ _ _ _ _ _ _ _ _ _ _ _]
      tunnel: w32 -> [w40 w179 w184 w202 w208 w213 w217 w236 w242 w246 w252 w262 w273 w299 w304 w314 w318 w330 w343 w356 w369 w382 w400 w415 w430 w445]
      tunnel: w31 -> [_ _ _ _ _ _ _ _ _ _ _ w257 w267 _ _ _ _ _ _ _ _ _ _ _ _ _]
      tunnel: w25 -> [w38 w176 w182 w193 w205 w211 w214 _ w237 w243 w250 w260 w269 w296 w301 w311 w315 w322 w337 w351 w364 w379 w394 w409 w424 w439]
      tunnel: [w37 w177 w186 w199 errorcluster {"status"=FALSE, "code"=0, "source"=""} ("error out") w210 w215 w233 w238 w244 w248 w258 w270 w297 w302 w312 w316 w328 w338 w347 w365 w376 w395 w410 w425 w440] -> w29
      tunnel: w23 -> [w36 w177 w185 w199 w204 w210 w215 w233 w239 w244 w249 w259 w271 w297 w302 w312 w316 w328 w339 w348 w366 w377 w396 w411 w426 w441]
      tunnel: [w39 w178 w183 w201 w207 w212 w216 w235 w241 w245 w251 w261 w272 w298 w303 w313 w317 w329 w342 w355 w368 w381 w399 w414 w429 w444] -> w28
      tunnel: [_ _ _ _ _ TRUE _ _ _ _ _ _ _ _ _ _ _ _ _ _ _ _ _ _ _ _] -> w27
      tunnel: [w35 w176 w182 w200 w205 w211 w214 w234 w237 w243 w250 w260 w269 w296 w301 w311 w315 w321 w337 w351 w364 w379 w393 w408 w423 w438] -> w26
      tunnel: w24 -> [w34 _ _ _ _ _ _ _ _ _ _ _ _ _ _ _ _ _ _ _ _ _ _ _ _ _]
      frame "", "Idle" {
        n23 = event shown="[2] \"Read Previous (Station B)\": Value Change" {
          selector: _ -> [_ _ _ _ _ _ _]
          dyn-events: _ -> [_ _ _ _ _ _ _]
          timeout: w34 -> [_ _ _ _ _ _ _]
          tunnel: w40 -> [w44 w67 w93 w119 w144 w169 w175]
          tunnel: [w43 w66 w92 w118 w143 w168 w174] -> w39
          tunnel: w38 -> [w41 w56 w82 w108 w133 w162 w172]
          tunnel: [w42 w59 w85 w111 w136 w160 w173] -> w37
          tunnel: w36 -> [w42 w53 w79 w105 w130 w166 w173]
          tunnel: [w41 w58 w84 w110 w135 w161 w172] -> w35
          event Timeout {
            n24 = event-data() -> ()  [unwired: 1 in, 1 out]
            n25 = call <vilib>:"Add State(s) to Queue__jki_lib_state_machine.vi"("State(s) in (\"\")"=w44) -> ("States Out"=w43:string)  [unwired: 14 in]
          }
          event "Read Previous (Station A)": Value Change {
            # "If the history file\ndoes not have all\nof the values it creates\nnew files all the time\nThis populates and \nensures everything \nis entered correctly"
            n26 = event-data() -> ()  [unwired: 1 in, 6 out]
            n27 = Unbundle By Name(w56) -> ("File Locations In (Station A)"=w54:T4)
            n28 = call "HCC Read Write Display.vi"(6:TRUE ("Active Station"), "Read Write Control"=enum16{"Read", "Write"}."Read", "error in (no error)"=w53, 9:"A" ("Station ID"), "File Locations In"=w54) -> ("error out"=w48:errorcluster, "Washer Output"=w57:T6, 3:w47)  [unwired: 4 in]
            n29 = local read "Front Panel (Station A)"() -> ()  [unwired: 1 in]
            n30 = Unbundle By Name() -> ("Serial Number"=w51:string, "Lab ID"=w50:string, "TR Number"=w49:string)  [unwired: 1 in]
            n31 = Bundle By Name(cluster=w56, "File Locations In (Station A)"=w47, "Main Washer Control (Station A)"=w57) -> (w58:T17)
            n32 = Equal?(x=w50, y="") -> (x = y?=w62:bool)
            n33 = Equal?(x=w49, y="") -> (x = y?=w61:bool)
            n34 = Equal?(x=w51, y="") -> (x = y?=w63:bool)
            n35 = Compound Arithmetic op=AND(w63, w62, w61) -> (w60:bool)
            n36 = case shown="True" w60 {
              tunnel: w48 -> [w68 w69]
              tunnel: [w68 w69] -> w59
              frame False {
              }
              frame True {
                n37 = One Button Dialog(message="No History File Found!") -> ()  [unwired: 1 in, 1 out]
              }
            }
            n38 = call <vilib>:"Add State(s) to Queue__jki_lib_state_machine.vi"("State(s) in (\"\")"=w67) -> ("States Out"=w66:string)  [unwired: 14 in]
          }
          event "Read Previous (Station B)": Value Change {
            # "If the history file\ndoes not have all\nof the values it creates\nnew files all the time\nThis populates and \nensures everything \nis entered correctly"
            n39 = event-data() -> ()  [unwired: 1 in, 6 out]
            n40 = Unbundle By Name(w82) -> ("File Locations In (Station A)"=w80:T4)
            n41 = call "HCC Read Write Display.vi"(6:TRUE ("Active Station"), "Read Write Control"=enum16{"Read", "Write"}."Read", "error in (no error)"=w79, 9:"B" ("Station ID"), "File Locations In"=w80) -> ("error out"=w74:errorcluster, "Washer Output"=w83:T6, 3:w73)  [unwired: 4 in]
            n42 = Unbundle By Name() -> ("Serial Number"=w77:string, "Lab ID"=w76:string, "TR Number"=w75:string)  [unwired: 1 in]
            n43 = local read "Front Panel (Station B)"() -> ()  [unwired: 1 in]
            n44 = Bundle By Name(cluster=w82, "File Locations In (Station B)"=w73, "Main Washer Control (Station B)"=w83) -> (w84:T17)
            n45 = Equal?(x=w76, y="") -> (x = y?=w88:bool)
            n46 = Equal?(x=w75, y="") -> (x = y?=w87:bool)
            n47 = Equal?(x=w77, y="") -> (x = y?=w89:bool)
            n48 = Compound Arithmetic op=AND(w89, w88, w87) -> (w86:bool)
            n49 = case shown="True" w86 {
              tunnel: w74 -> [w94 w95]
              tunnel: [w94 w95] -> w85
              frame False {
              }
              frame True {
                n50 = One Button Dialog(message="No History File Found!") -> ()  [unwired: 1 in, 1 out]
              }
            }
            n51 = call <vilib>:"Add State(s) to Queue__jki_lib_state_machine.vi"("State(s) in (\"\")"=w93) -> ("States Out"=w92:string)  [unwired: 14 in]
          }
          event "Read Previous (Station C)": Value Change {
            # "If the history file\ndoes not have all\nof the values it creates\nnew files all the time\nThis populates and \nensures everything \nis entered correctly"
            n52 = event-data() -> ()  [unwired: 1 in, 6 out]
            n53 = Unbundle By Name(w108) -> ("File Locations In (Station A)"=w106:T4)
            n54 = call "HCC Read Write Display.vi"(6:TRUE ("Active Station"), "Read Write Control"=enum16{"Read", "Write"}."Read", "error in (no error)"=w105, 9:"C" ("Station ID"), "File Locations In"=w106) -> ("error out"=w100:errorcluster, "Washer Output"=w109:T6, 3:w99)  [unwired: 4 in]
            n55 = Unbundle By Name() -> ("Serial Number"=w103:string, "Lab ID"=w102:string, "TR Number"=w101:string)  [unwired: 1 in]
            n56 = Bundle By Name(cluster=w108, "File Locations In (Station C)"=w99, "Main Washer Control (Station C)"=w109) -> (w110:T17)
            n57 = local read "Front Panel (Station C)"() -> ()  [unwired: 1 in]
            n58 = Equal?(x=w102, y="") -> (x = y?=w114:bool)
            n59 = Equal?(x=w101, y="") -> (x = y?=w113:bool)
            n60 = Equal?(x=w103, y="") -> (x = y?=w115:bool)
            n61 = Compound Arithmetic op=AND(w115, w114, w113) -> (w112:bool)
            n62 = case shown="True" w112 {
              tunnel: w100 -> [w120 w121]
              tunnel: [w120 w121] -> w111
              frame False {
              }
              frame True {
                n63 = One Button Dialog(message="No History File Found!") -> ()  [unwired: 1 in, 1 out]
              }
            }
            n64 = call <vilib>:"Add State(s) to Queue__jki_lib_state_machine.vi"("State(s) in (\"\")"=w119) -> ("States Out"=w118:string)  [unwired: 14 in]
          }
          event "Read Previous (Station D)": Value Change {
            (unwired) TRUE ("Active Station")
            # "If the history file\ndoes not have all\nof the values it creates\nnew files all the time\nThis populates and \nensures everything \nis entered correctly"
            n65 = event-data() -> ()  [unwired: 1 in, 6 out]
            n66 = Unbundle By Name(w133) -> ("File Locations In (Station A)"=w131:T4)
            n67 = call "HCC Read Write Display.vi"("Read Write Control"=enum16{"Read", "Write"}."Read", "error in (no error)"=w130, 9:"D" ("Station ID"), "File Locations In"=w131) -> ("error out"=w125:errorcluster, "Washer Output"=w134:T6, 3:w124)  [unwired: 5 in]
            n68 = Unbundle By Name() -> ("Serial Number"=w128:string, "Lab ID"=w127:string, "TR Number"=w126:string)  [unwired: 1 in]
            n69 = Bundle By Name(cluster=w133, "File Locations In (Station D)"=w124, "Main Washer Control (Station D)"=w134) -> (w135:T17)
            n70 = local read "Front Panel (Station D)"() -> ()  [unwired: 1 in]
            n71 = Equal?(x=w127, y="") -> (x = y?=w139:bool)
            n72 = Equal?(x=w126, y="") -> (x = y?=w138:bool)
            n73 = Equal?(x=w128, y="") -> (x = y?=w140:bool)
            n74 = Compound Arithmetic op=AND(w140, w139, w138) -> (w137:bool)
            n75 = case shown="True" w137 {
              tunnel: w125 -> [w145 w146]
              tunnel: [w145 w146] -> w136
              frame False {
              }
              frame True {
                n76 = One Button Dialog(message="No History File Found!") -> ()  [unwired: 1 in, 1 out]
              }
            }
            n77 = call <vilib>:"Add State(s) to Queue__jki_lib_state_machine.vi"("State(s) in (\"\")"=w144) -> ("States Out"=w143:string)  [unwired: 14 in]
          }
          event "Complete": Value Change {
            # "Get the latest data from the user"
            n78 = event-data() -> ()  [unwired: 1 in, 1 out]
            n79 = Unbundle By Name(w162) -> ("Main Washer Control (Station D)"=w156:T6, "Main Washer Control (Station C)"=w157:T6, "Main Washer Control (Station B)"=w158:T6, "Main Washer Control (Station A)"=w159:T6)
            n80 = local read "Front Panel (Station D)"() -> (w151:T2)
            n81 = local read "Front Panel (Station C)"() -> (w150:T2)
            n82 = local read "Front Panel (Station B)"() -> (w149:T2)
            n83 = local read "Front Panel (Station A)"() -> (w148:T2)
            n84 = call "Save File Get Latest Data.vi"("Front Panel In"=w148, "Error In"=w166, "Main Washer Control In"=w159) -> ("Error Out"=w163:errorcluster, "Main Washer Control Out"=w152:T6)  [unwired: 7 in]
            n85 = call "Save File Get Latest Data.vi"("Front Panel In"=w149, "Error In"=w163, "Main Washer Control In"=w158) -> ("Error Out"=w164:errorcluster, "Main Washer Control Out"=w153:T6)  [unwired: 7 in]
            n86 = call "Save File Get Latest Data.vi"("Front Panel In"=w150, "Error In"=w164, "Main Washer Control In"=w157) -> ("Error Out"=w165:errorcluster, "Main Washer Control Out"=w154:T6)  [unwired: 7 in]
            n87 = call "Save File Get Latest Data.vi"("Front Panel In"=w151, "Error In"=w165, "Main Washer Control In"=w156) -> ("Error Out"=w160:errorcluster, "Main Washer Control Out"=w155:T6)  [unwired: 7 in]
            n88 = Bundle By Name(cluster=w162, "Front Panel (Station D)"=w151, "Front Panel (Station C)"=w150, "Front Panel (Station B)"=w149, "Front Panel (Station A)"=w148, "Main Washer Control (Station D)"=w155, "Main Washer Control (Station C)"=w154, "Main Washer Control (Station B)"=w153, "Main Washer Control (Station A)"=w152) -> (w161:T17)
            n89 = call <vilib>:"Add State(s) to Queue__jki_lib_state_machine.vi"("State(s) in Front (\"\")"="Check Active Station", "State(s) in (\"\")"=w169) -> ("States Out"=w168:string)  [unwired: 13 in]
          }
          event Panel Close? {
            n90 = event-data() -> ()  [unwired: 1 in, 1 out]
            n91 = event-data("Discard?"=TRUE) -> ()  [unwired: 1 in, 1 out]
            n92 = call <vilib>:"Add State(s) to Queue__jki_lib_state_machine.vi"("State(s) in Front (\"\")"="Macro: Exit", "State(s) in (\"\")"=w175) -> ("States Out"=w174:string)  [unwired: 13 in]
          }
        }
      }
      frame "---------- Core ----------" {
        n93 = call <vilib>:"Add State(s) to Queue__jki_lib_state_machine.vi"("State(s) in (\"\")"=w179) -> ("States Out"=w178:string)  [unwired: 14 in]
      }
      frame Default {
        w189 = 42 items=["No error", "Argument error", "Memory is full", "Out of zone", "End of file", "File already open", "Generic file I/O error", "File not found", "File permission error", "Disk is full", "Duplicate path", "Too many files open", "System feature not enabled", "Resource file not found", "Cannot add resource", "Resource not found", "Image not found", "Image memory error", "Pen does not exist", "Config type invalid", "Config token not found", "Config parse error", "Config memory error", "Bad external code format", "Bad external code offset", "External code not present", "Null window", "Destroy window error", "Null menu", "Print aborted", "Bad print record", "Print driver error", "Windows error during printing", "Memory error during printing", "Print dialog error", "Generic print error", "Invalid device refnum", "Device not found", "Device parameter error", "Device unit error", "Cannot open device", "Device call aborted", "Generic error", "Cancelled by user", "Object ID too low", "Object ID too high", "Object not in heap", "Unknown heap", "Unknown object (invalid DefProc)", "Unknown object (DefProc not in table)", "Message out of range", "Invalid (null) method", "Unknown message", "Manager call not supported", "Bad address", "Network operation in progress", "Network operation timed out", "Connection is busy", "Network attribute not supported", "Network error", "Address in use", "System out of memory", "Connection aborted", "Connection refused", "Not connected", "Already connected", "Connection closed", "Initialization error (interapplication manager)", "Bad occurrence", "Wait on unbound occurrence handler", "Occurrence queue overflow", "Datalog type conflict", "Unused", "Unrecognized type (interapplication manager)", "Memory corrupt", "Failed to make temporary DLL", "Old CIN version", "Drag socket not found", "Failed to load drop-object", "Failed to register OLE object", "Failed to release OLE object", "Format specifier type mismatch", "Unknown format specifier", "Too few format specifiers", "Too many format specifiers", "Scan failed", "Newer CIN version", "Error converting to variant", "Runtime menu error", "Password tampered", "Variant attribute not found", "Incompatible variant data type", "Event data is not available", "Event Store is not present", "Occurrence is not found", "Event Queue is not created", "Event info is not available", "Refnum passed is NULL", "Error retrieving Class GUID", "Error retrieving CoClass GUID", "Error retrieving TypeLib GUID.", "Bad built application magic bytes.", "Specific driver is different from the specific driver associated with the Logical Name.", "There is no session opened to the class driver.", "Max Error", "MAX - Error with config objects", "MAX - Error loading configuration", "MAX - Group not supported"]
        # "Current State"
        # "Handle mistyped state name (developer tool)"
        n94 = Format Into String(format string="Software Exception: Unhandled State \"%s\"." ("message"), error in=w185, w180) -> (resulting string=w188:string, error out=w187:errorcluster)  [unwired: 1 in]
        n95 = call <vilib>:"Error Cluster From Error Code.vi"("show call chain? (False)"=TRUE, "error in (no error)"=w187, "error message (\"\")"=w188, "error code (0)"=w189) -> ("error out"=w186:errorcluster)  [unwired: 5 in]
        n96 = call <vilib>:"Add State(s) to Queue__jki_lib_state_machine.vi"("State(s) in (\"\")"=w184) -> ("States Out"=w183:string)  [unwired: 14 in]
      }
      frame "Initialize Core Data" {
        # "originally closed?"
        # "exe?"
        # "If panel starts closed or is an EXE, then close it when we exit"
        n97 = property class="VI"() -> ("Front Panel.Open"=w198:bool)  [unwired: 2 in, 2 out]
        n98 = property class="App"() -> ("App.Kind"=w197:T15)  [unwired: 2 in, 2 out]
        n99 = control-ref of="Current VI Reference"() -> (w191:refnum<vi>)
        n100 = Not(x=w198) -> (.not. x?=w195:bool)
        n101 = Equal?(x=w197, y=T15."Run Time System" ("Application:Kind")) -> (x = y?=w194:bool)
        n102 = Or(x=w195, y=w194) -> (x .or. y?=w192:bool)
        n103 = Bundle By Name(cluster=w193, "Core.Current VI Reference"=w191, "Core.Close Panel on Exit?"=w192) -> (w200:T17)
        n104 = call <vilib>:"Add State(s) to Queue__jki_lib_state_machine.vi"("State(s) in (\"\")"=w202) -> ("States Out"=w201:string)  [unwired: 14 in]
      }
      frame "Error Handler" {
        # "Unhandled Error -- Display it"
        # "Clear error"
        n105 = call <vilib>:"General Error Handler.vi"("error in (no error)"=w204) -> ()  [unwired: 10 in, 5 out]
        n106 = call <vilib>:"Add State(s) to Queue__jki_lib_state_machine.vi"("State(s) in Front (\"\")"="/* Post Error States", "State(s) in (\"\")"=w208) -> ("States Out"=w207:string)  [unwired: 13 in]
      }
      frame "Exit" {
        n107 = call <vilib>:"Add State(s) to Queue__jki_lib_state_machine.vi"("State(s) in (\"\")"=w213) -> ("States Out"=w212:string)  [unwired: 14 in]
      }
      frame "---------- Data ----------" {
        n108 = call <vilib>:"Add State(s) to Queue__jki_lib_state_machine.vi"("State(s) in (\"\")"=w217) -> ("States Out"=w216:string)  [unwired: 14 in]
      }
      frame "Data: Initialize" {
        w219 = bool[] [FALSE, FALSE, FALSE, FALSE]  # Active Stations
        w232 = T18 {"Current VI Reference"=refnum, "Close Panel on Exit?"=FALSE}  # Core
        n109 = call <vilib>:"Add State(s) to Queue__jki_lib_state_machine.vi"("State(s) in (\"\")"=w236) -> ("States Out"=w235:string)  [unwired: 14 in]
        n110 = Bundle("Core"=w232, "Main Washer Control (Station A)"="Main Washer Control (Station A)", "Main Washer Control (Station B)"="Main Washer Control (Station B)", "Main Washer Control (Station C)"="Main Washer Control (Station C)", "Main Washer Control (Station D)"="Main Washer Control (Station D)", "Front Panel (Station A)"="Front Panel (Station A)", "Front Panel (Station B)"="Front Panel (Station B)", "Front Panel (Station C)"="Front Panel (Station C)", "Front Panel (Station D)"="Front Panel (Station D)", "File Locations In (Station A)"="File Locations In (Station A)", "File Locations In (Station B)"="File Locations In (Station B)", "File Locations In (Station C)"="File Locations In (Station C)", "File Locations In (Station D)"="File Locations In (Station D)", "Active Stations"=w219, "RLT Station Type"="RLT Station Type") -> (w234:T17)  [unwired: 1 in]
      }
      frame "Data: Cleanup" {
        n111 = Unbundle By Name(w237) -> ("Core.Current VI Reference"=w240:refnum<vi>)
        n112 = Close Reference(reference=w240, error in (no error)=w239) -> (error out=w238:errorcluster)
        n113 = call <vilib>:"Add State(s) to Queue__jki_lib_state_machine.vi"("State(s) in (\"\")"=w242) -> ("States Out"=w241:string)  [unwired: 14 in]
      }
      frame "---------- UI ----------" {
        n114 = call <vilib>:"Add State(s) to Queue__jki_lib_state_machine.vi"("State(s) in (\"\")"=w246) -> ("States Out"=w245:string)  [unwired: 14 in]
      }
      frame "UI: Initialize" {
        n115 = Unbundle By Name(w250) -> ("RLT Station Type"=w247:T13)
        n116 = case shown="\"Single Station\", Default" w247 {
          tunnel: w249 -> [w253 w256]
          tunnel: [w253 w256] -> w248
          frame "Single Station", Default {
            w254 = T14."Disabled and Grayed Out" ("Disabled")
            w255 = T14."Disabled and Grayed Out" ("Disabled")
            n117 = property on="Read Previous (Station B)" class="Bool"("DisabledEnum"=w255) -> ()  [unwired: 2 in, 2 out]
            n118 = property on="Station B Check" class="Bool (strict)"("DisabledEnum"=w255) -> ()  [unwired: 2 in, 2 out]
            n119 = property on="Front Panel (Station B)" class="Clust (strict)"("DisabledEnum"=w255) -> ()  [unwired: 2 in, 2 out]
            n120 = property on="Read Previous (Station D)" class="Bool"("DisabledEnum"=w255) -> ()  [unwired: 2 in, 2 out]
            n121 = property on="Station D Check" class="Bool (strict)"("DisabledEnum"=w255) -> ()  [unwired: 2 in, 2 out]
            n122 = property on="Front Panel (Station D)" class="Clust (strict)"("DisabledEnum"=w255) -> ()  [unwired: 2 in, 2 out]
            n123 = property on="Station C Check" class="Bool (strict)"("DisabledEnum"=w254) -> ()  [unwired: 2 in, 2 out]
            n124 = property on="Front Panel (Station C)" class="Clust (strict)"("DisabledEnum"=w254) -> ()  [unwired: 2 in, 2 out]
            n125 = property on="Read Previous (Station C)" class="Bool"("DisabledEnum"=w254) -> ()  [unwired: 2 in, 2 out]
          }
          frame "Four Stations" {
          }
        }
        n126 = call <vilib>:"Add State(s) to Queue__jki_lib_state_machine.vi"("State(s) in (\"\")"=w252) -> ("States Out"=w251:string)  [unwired: 14 in]
      }
      frame "UI: Cursor Set" {
        # "Argument"
        n127 = case shown="\"Idle\", Default" w257 {
          tunnel: w259 -> [w264 w266]
          tunnel: [w263 w265] -> w258
          frame "Idle", Default {
            n128 = call <vilib>:"Unset Busy.vi"("error in (no error)"=w264) -> ("error out"=w263:errorcluster)  [unwired: 10 in]
          }
          frame "Busy" {
            n129 = call <vilib>:"Set Busy.vi"("error in (no error)"=w266) -> ("error out"=w265:errorcluster)  [unwired: 9 in, 1 out]
          }
        }
        n130 = call <vilib>:"Add State(s) to Queue__jki_lib_state_machine.vi"("State(s) in (\"\")"=w262) -> ("States Out"=w261:string)  [unwired: 14 in]
      }
      frame "UI: Front Panel State" {
        # "Argument"
        n131 = Unbundle By Name(w269) -> ("Core.Current VI Reference"=w268:refnum<vi>)
        n132 = case shown="\"Open\", Default" w267 {
          tunnel: w271 -> [w277 w290]
          tunnel: [w279 w291] -> w270
          tunnel: w268 -> [w278 w288]
          frame "Open", Default {
            n133 = property class="VI"(reference=w278, error in=w277) -> (reference out=w275:refnum<vi>, error out=w276:errorcluster, "Front Panel.Open"=w274:bool)
            n134 = case shown="False" w274 {
              tunnel: [w282 w285] -> w279
              tunnel: w276 -> [w281 w285]
              tunnel: w275 -> [w280 _]
              frame False {
                n135 = invoke class="VI" method="FP.Open"(reference=w280, error in=w281, "Activate"=TRUE, "State"=T16."Standard") -> (error out=w282:errorcluster)  [unwired: 1 in, 4 out]
              }
              frame True {
              }
            }
          }
          frame "Close" {
            n136 = property class="VI"(reference=w288, error in=w290) -> (reference out=w287:refnum<vi>, error out=w289:errorcluster, "Front Panel.Open"=w286:bool)
            n137 = case shown="True" w286 {
              tunnel: [w292 w295] -> w291
              tunnel: w289 -> [w292 w294]
              tunnel: w287 -> [_ w293]
              frame False {
              }
              frame True {
                n138 = invoke class="VI" method="FP.Close"(reference=w293, error in=w294) -> (error out=w295:errorcluster)  [unwired: 1 in, 2 out]
              }
            }
          }
        }
        n139 = call <vilib>:"Add State(s) to Queue__jki_lib_state_machine.vi"("State(s) in (\"\")"=w273) -> ("States Out"=w272:string)  [unwired: 14 in]
      }
      frame "---------- Macro ----------" {
        n140 = call <vilib>:"Add State(s) to Queue__jki_lib_state_machine.vi"("State(s) in (\"\")"=w299) -> ("States Out"=w298:string)  [unwired: 14 in]
      }
      frame "Macro: Initialize" {
        w300 = "Data: Initialize\nInitialize Core Data\nUI: Initialize\nUI: Front Panel State >> Open"  # Data: Initialize Initialize Core Data UI: Initialize UI: Front Panel State >> Open
        n141 = call <vilib>:"Add State(s) to Queue__jki_lib_state_machine.vi"("State(s) in Front (\"\")"=w300, "State(s) in (\"\")"=w304) -> ("States Out"=w303:string)  [unwired: 13 in]
      }
      frame "Macro: Exit" {
        n142 = Unbundle By Name(w311) -> ("Core.Close Panel on Exit?"=w310:bool)
        n143 = Select(t="UI: Front Panel State >> Close", s=w310, f="") -> (s? t:f=w307:string)
        n144 = call <vilib>:"Add State(s) to Queue__jki_lib_state_machine.vi"("State(s) in (\"\")"=w307, "State(s) at Back (\"\")"="Data: Cleanup\nExit") -> ("States Out"=w305:string)  [unwired: 13 in]
        n145 = call <vilib>:"Add State(s) to Queue__jki_lib_state_machine.vi"("State(s) in Front (\"\")"=w305, "State(s) in (\"\")"=w314) -> ("States Out"=w313:string)  [unwired: 13 in]
      }
      frame "----------File Name Setup ----------" {
        n146 = call <vilib>:"Add State(s) to Queue__jki_lib_state_machine.vi"("State(s) in (\"\")"=w318) -> ("States Out"=w317:string)  [unwired: 14 in]
      }
      frame "Check Active Station" {
        n147 = Build Array("Station A Check", "Station B Check", "Station C Check", "Station D Check") -> (w320:bool[])
        n148 = Or Array Elements(Boolean array=w320) -> (logical OR=w327:bool)
        n149 = case shown="True" w327 {
          tunnel: ["" "Check for Blanks Station A"] -> w319
          frame False {
            n150 = One Button Dialog(message="No Active Station Selected") -> ()  [unwired: 1 in, 1 out]
          }
          frame True {
          }
        }
        n151 = Bundle By Name(cluster=w322, "Active Stations"=w320) -> (w321:T17)
        n152 = call <vilib>:"Add State(s) to Queue__jki_lib_state_machine.vi"("State(s) in Front (\"\")"=w319, "State(s) in (\"\")"=w330) -> ("States Out"=w329:string)  [unwired: 13 in]
      }
      frame "Check for Blanks Station A" {
        n153 = Unbundle By Name(w337) -> ("Front Panel (Station A)"=w336:T2, "Active Stations"=w335:bool[])
        n154 = call "Save File Check For Blanks.vi"("Error In"=w339, "Station Index"=0 ("index"), "Active Stations"=w335, "Front Panel In"=w336) -> ("Error Out"=w338:errorcluster, "Blanks (T)"=w340:bool)  [unwired: 6 in]
        n155 = case shown="False" w340 {
          tunnel: ["Check for Blanks Station B" ""] -> w341
          frame False {
          }
          frame True {
            n156 = One Button Dialog(message="Fill out:\nSerial Number\nLab ID\nTR Number\nUnit Type") -> ()  [unwired: 1 in, 1 out]
          }
        }
        n157 = call <vilib>:"Add State(s) to Queue__jki_lib_state_machine.vi"("State(s) in Front (\"\")"=w341, "State(s) in (\"\")"=w343) -> ("States Out"=w342:string)  [unwired: 13 in]
      }
      frame "Check for Blanks Station B" {
        n158 = Unbundle By Name(w351) -> ("Front Panel (Station B)"=w349:T2, "Active Stations"=w350:bool[])
        n159 = call "Save File Check For Blanks.vi"("Error In"=w348, "Station Index"=1 ("index"), "Active Stations"=w350, "Front Panel In"=w349) -> ("Error Out"=w347:errorcluster, "Blanks (T)"=w353:bool)  [unwired: 6 in]
        n160 = case shown="False" w353 {
          tunnel: ["Check for Blanks Station C" ""] -> w354
          frame False {
          }
          frame True {
            n161 = One Button Dialog(message="Fill out:\nSerial Number\nLab ID\nTR Number\nUnit Type") -> ()  [unwired: 1 in, 1 out]
          }
        }
        n162 = call <vilib>:"Add State(s) to Queue__jki_lib_state_machine.vi"("State(s) in Front (\"\")"=w354, "State(s) in (\"\")"=w356) -> ("States Out"=w355:string)  [unwired: 13 in]
      }
      frame "Check for Blanks Station C" {
        n163 = Unbundle By Name(w364) -> ("Front Panel (Station C)"=w363:T2, "Active Stations"=w362:bool[])
        n164 = call "Save File Check For Blanks.vi"("Error In"=w366, "Station Index"=2 ("index"), "Active Stations"=w362, "Front Panel In"=w363) -> ("Error Out"=w365:errorcluster, "Blanks (T)"=w360:bool)  [unwired: 6 in]
        n165 = case shown="False" w360 {
          tunnel: ["Check for Blanks Station D" ""] -> w367
          frame False {
          }
          frame True {
            n166 = One Button Dialog(message="Fill out:\nSerial Number\nLab ID\nTR Number\nUnit Type") -> ()  [unwired: 1 in, 1 out]
          }
        }
        n167 = call <vilib>:"Add State(s) to Queue__jki_lib_state_machine.vi"("State(s) in Front (\"\")"=w367, "State(s) in (\"\")"=w369) -> ("States Out"=w368:string)  [unwired: 13 in]
      }
      frame "Check for Blanks Station D" {
        n168 = Unbundle By Name(w379) -> ("Front Panel (Station D)"=w378:T2, "Active Stations"=w375:bool[])
        n169 = call "Save File Check For Blanks.vi"("Error In"=w377, "Station Index"=3 ("index"), "Active Stations"=w375, "Front Panel In"=w378) -> ("Error Out"=w376:errorcluster, "Blanks (T)"=w374:bool)  [unwired: 6 in]
        n170 = case shown="False" w374 {
          tunnel: ["Update Backup File Station A\nUpdate Backup File Station B\nUpdate Backup File Station C\nUpdate Backup File Station D\nMacro: Exit" ""] -> w380
          frame False {
          }
          frame True {
            n171 = One Button Dialog(message="Fill out:\nSerial Number\nLab ID\nTR Number\nUnit Type") -> ()  [unwired: 1 in, 1 out]
          }
        }
        n172 = call <vilib>:"Add State(s) to Queue__jki_lib_state_machine.vi"("State(s) in Front (\"\")"=w380, "State(s) in (\"\")"=w382) -> ("States Out"=w381:string)  [unwired: 13 in]
      }
      frame "Update Backup File Station A" {
        n173 = Unbundle By Name(w394) -> ("File Locations In (Station A)"=w398:T4, "Main Washer Control (Station A)"=w397:T6, "Active Stations"=w390:bool[])
        n174 = Index Array(array=w390, index=0) -> (element=w386:bool)
        n175 = call "HCC Read Write Display.vi"(6:w386, "Read Write Control"=enum16{"Read", "Write"}."Write", "error in (no error)"=w396, 9:"A" ("Station ID"), "Washer Input"=w397, "File Locations In"=w398) -> ("error out"=w395:errorcluster, "Washer Output"=w391:T6, 3:w392)  [unwired: 3 in]
        n176 = Bundle By Name(cluster=w394, "File Locations In (Station A)"=w392, "Main Washer Control (Station A)"=w391) -> (w393:T17)
        n177 = call <vilib>:"Add State(s) to Queue__jki_lib_state_machine.vi"("State(s) in (\"\")"=w400) -> ("States Out"=w399:string)  [unwired: 14 in]
      }
      frame "Update Backup File Station B" {
        n178 = Unbundle By Name(w409) -> ("File Locations In (Station A)"=w413:T4, "Main Washer Control (Station B)"=w412:T6, "Active Stations"=w404:bool[])
        n179 = Index Array(array=w404, index=1) -> (element=w401:bool)
        n180 = call "HCC Read Write Display.vi"(6:w401, "Read Write Control"=enum16{"Read", "Write"}."Write", "error in (no error)"=w411, 9:"B" ("Station ID"), "Washer Input"=w412, "File Locations In"=w413) -> ("error out"=w410:errorcluster, "Washer Output"=w406:T6, 3:w407)  [unwired: 3 in]
        n181 = Bundle By Name(cluster=w409, "File Locations In (Station B)"=w407, "Main Washer Control (Station B)"=w406) -> (w408:T17)
        n182 = call <vilib>:"Add State(s) to Queue__jki_lib_state_machine.vi"("State(s) in (\"\")"=w415) -> ("States Out"=w414:string)  [unwired: 14 in]
      }
      frame "Update Backup File Station C" {
        n183 = Unbundle By Name(w424) -> ("File Locations In (Station A)"=w428:T4, "Main Washer Control (Station C)"=w427:T6, "Active Stations"=w419:bool[])
        n184 = Index Array(array=w419, index=2) -> (element=w416:bool)
        n185 = call "HCC Read Write Display.vi"(6:w416, "Read Write Control"=enum16{"Read", "Write"}."Write", "error in (no error)"=w426, 9:"C" ("Station ID"), "Washer Input"=w427, "File Locations In"=w428) -> ("error out"=w425:errorcluster, "Washer Output"=w421:T6, 3:w422)  [unwired: 3 in]
        n186 = Bundle By Name(cluster=w424, "File Locations In (Station C)"=w422, "Main Washer Control (Station C)"=w421) -> (w423:T17)
        n187 = call <vilib>:"Add State(s) to Queue__jki_lib_state_machine.vi"("State(s) in (\"\")"=w430) -> ("States Out"=w429:string)  [unwired: 14 in]
      }
      frame "Update Backup File Station D" {
        n188 = Unbundle By Name(w439) -> ("File Locations In (Station A)"=w443:T4, "Main Washer Control (Station D)"=w442:T6, "Active Stations"=w434:bool[])
        n189 = Index Array(array=w434, index=3) -> (element=w431:bool)
        n190 = call "HCC Read Write Display.vi"(6:w431, "Read Write Control"=enum16{"Read", "Write"}."Write", "error in (no error)"=w441, 9:"D" ("Station ID"), "Washer Input"=w442, "File Locations In"=w443) -> ("error out"=w440:errorcluster, "Washer Output"=w436:T6, 3:w437)  [unwired: 3 in]
        n191 = Bundle By Name(cluster=w439, "File Locations In (Station D)"=w437, "Main Washer Control (Station D)"=w436) -> (w438:T17)
        n192 = call <vilib>:"Add State(s) to Queue__jki_lib_state_machine.vi"("State(s) in (\"\")"=w445) -> ("States Out"=w444:string)  [unwired: 14 in]
      }
    }
  }
  "error out" <- w16
  n193 = Unbundle By Name(w14) -> ("Main Washer Control (Station A)"=w9:T6, "Main Washer Control (Station B)"=w8:T6, "Main Washer Control (Station C)"=w7:T6, "Main Washer Control (Station D)"=w6:T6, "Active Stations"=→"Active Stations":bool[])
  n194 = Unbundle By Name(w14) -> ("File Locations In (Station A)"=w13:T4, "File Locations In (Station B)"=w12:T4, "File Locations In (Station C)"=w11:T4, "File Locations In (Station D)"=w10:T4)
  n195 = Build Array(w9, w8, w7, w6) -> (→"Main Washer Controls Out":T6[])
  n196 = Build Array(w13, w12, w11, w10) -> (→"File Locations Out":T4[])
